vi "Playloop_Length--Const.vi"() -> (3 "AWG Length Command":string)   [LabVIEW 2017, in "Communications Library.lvlib"]
uses:
  Communications Library.lvlib
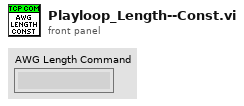
[diagram p1: front panel]
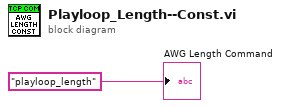
[diagram p0: block diagram]
diagram:
  "AWG Length Command" <- "playloop_length" ("data in")
